vi "IMyInterface2.MyInterfaceMethod.vi"(0 "reference in":refnum<class "MyClass4.lvclass">, 1 "MyParameter":dbl, 5 "error in (no error)":errorcluster) -> (14 "reference out":refnum<class "MyClass4.lvclass">, 19 "error out":errorcluster)   [LabVIEW 2017, in "MyClass4.lvclass"]
uses:
  MyClass4.lvclass
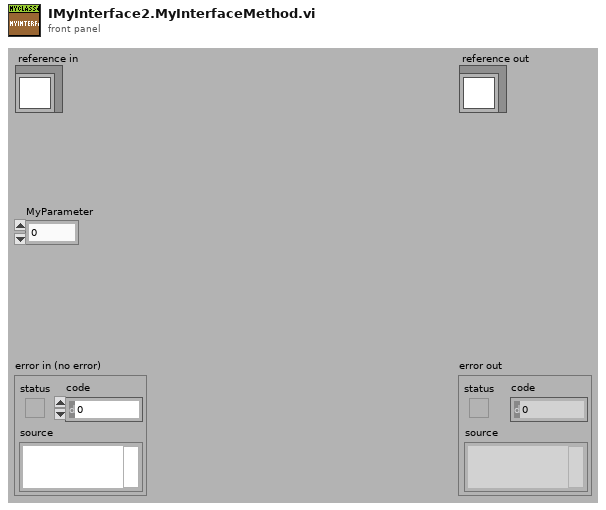
[diagram p1: front panel]
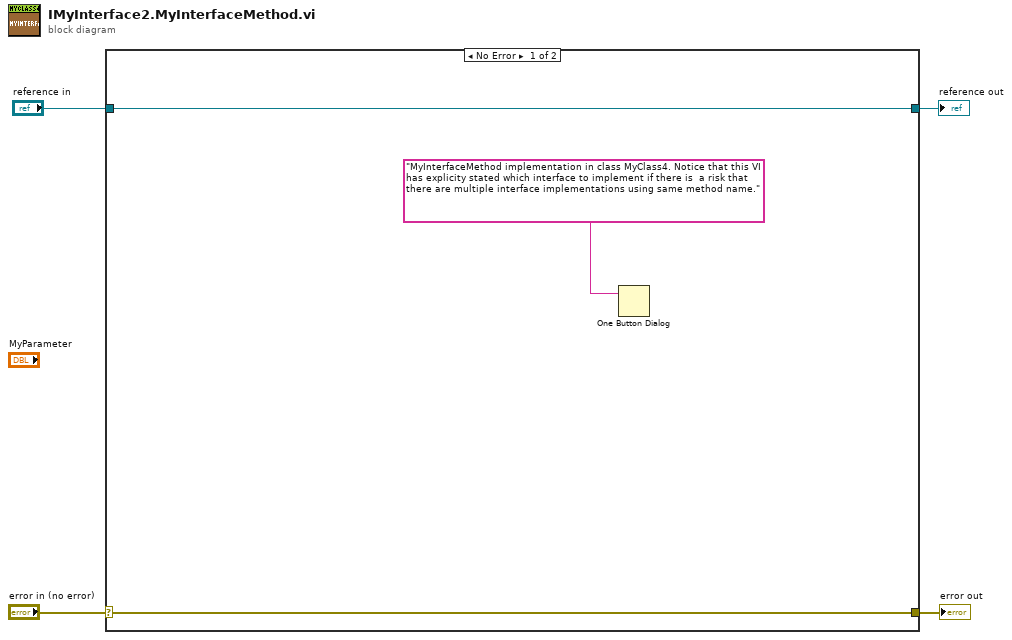
[diagram p0: block diagram]
diagram:
  n1 = case shown="No Error" "error in (no error)" {
    selector: "error in (no error)" -> [w6 w9]
    tunnel: [w6 w9] -> w3
    tunnel: [w7 w8] -> w1
    tunnel: "reference in" -> [w7 w8]
    frame No Error {
      n2 = One Button Dialog(message="MyInterfaceMethod implementation in class MyClass4. Notice that this VI has explicity stated which interface to implement if there is  a risk that there are multiple interface implementations using same method name.") -> ()  [unwired: 1 in, 1 out]
    }
    frame Error {
    }
  }
  "error out" <- w3
  "reference out" <- w1
